vi "clump to runtime maps.vi"(4 "output dictionary":refnum<class "data dictionary.lvclass">, 6 "input dictionary":refnum<class "data dictionary.lvclass">, 7 "modbus channels":refnum<class "Modbus Module Channel.lvclass">[](array[class]), 8 "error in":errorcluster, 11 "clumps":T1[](array[typedef])) -> (0 "error out":errorcluster, 2 "output accesses":T7[](array[typedef]), 3 "input accesses":T4[](array[typedef]))   [LabVIEW 2013, in "Modbus Slave runtime.lvclass"]
uses:
  Modbus Slave runtime.lvclass
  output bulk data access.ctl
  module channel/data bank type.ctl
  data mapping elements.ctl
  <vilib>/NI/Tag Bus/tag/Data Type.ctl
  bulk data access.ctl
  module channel/Modbus Module Channel.lvclass
  <vilib>/NI/Tag Bus/dictionary/data dictionary.lvclass
  clump.ctl
  <vilib>/NI/Tag Bus Module Framework/channel/channel classification.ctl
  <vilib>/NI/Tag Bus/tag/tag descriptor.lvclass/tag descriptor.ctl
  module channel/Modbus Module Channel.lvclass/Modbus Module Channel.ctl
  <vilib>/NI/Tag Bus/tag/read data type.vi
  module channel/Read starting address.vi
  module channel/Read subindex (bool).vi
  <vilib>/NI/Tag Bus/tag/read tag name.vi
  <vilib>/NI/Tag Bus/dictionary/locate tag.vi
  <vilib>/NI/Tag Bus/tag/tag descriptor.lvclass
  <vilib>/NI/Tag Bus Module Framework/channel/TBM channel.lvclass
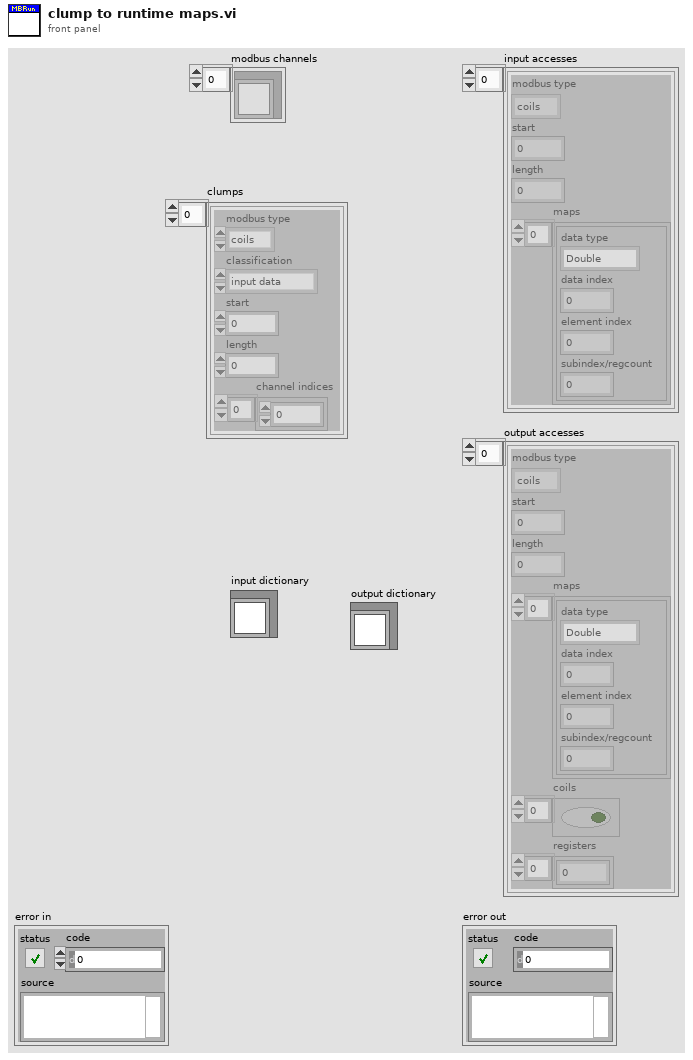
[diagram p1: front panel]
types:
  T1 = typedef "Modbus Slave runtime.lvclass/clump.ctl" = cluster{"modbus type":T2, "classification":T3, "start":i32, "length":i32, "channel indices":i32[]}
  T2 = typedef "Modbus Module Channel.lvclass/data bank type.ctl" = enum16{"coils", "discrete inputs", "input registers", "holding registers"}
  T3 = typedef "TBM channel.lvclass/channel classification.ctl" = enum16{"input data", "output data", "processing parameter", "processing result"}
  T4 = typedef "Modbus Slave runtime.lvclass/bulk data access.ctl" = cluster{"modbus type":T2, "start":u16, "length":u16, "maps":T5[]}
  T5 = typedef "Modbus Slave runtime.lvclass/data mapping elements.ctl" = cluster{"data type":T6, "data index":i32, "element index":i32, "subindex/regcount":i32}
  T6 = typedef "tag bus.lvlib/tag descriptor.lvclass/Data Type.ctl" = enum16{"Double", "Single", "I64", "I32", "I16", "I8", "U64", "U32", "U16", "U8", "Boolean", "String", "Array of Double", "Array of Single", "Array of I64", "Array of I32", "Array of I16", "Array of I8", "Array of U64", "Array of U32", "Array of U16", "Array of U8", "Array of Boolean", "Array of String"}
  T7 = typedef "Modbus Slave runtime.lvclass/output bulk data access.ctl" = cluster{"modbus type":T2, "start":u16, "length":u16, "maps":T5[], "coils":bool[], "registers":u16[]}
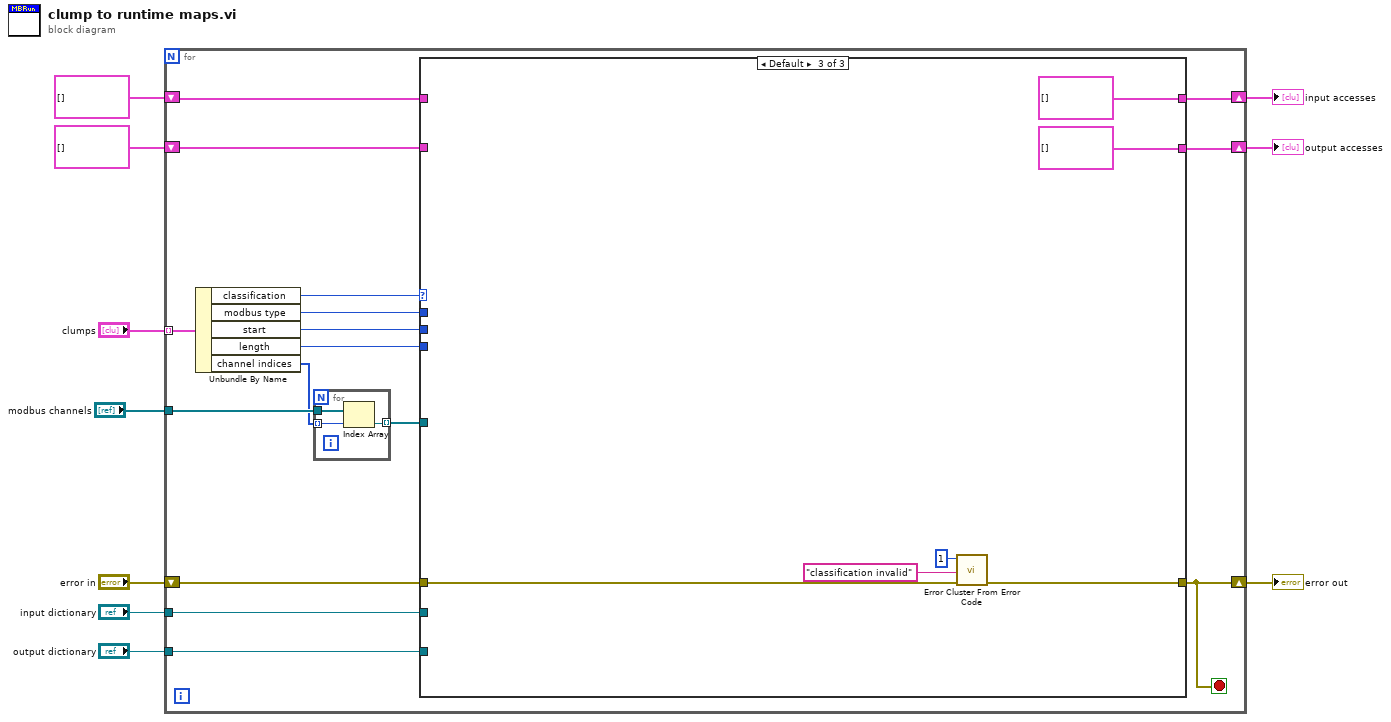
[diagram p0: block diagram]
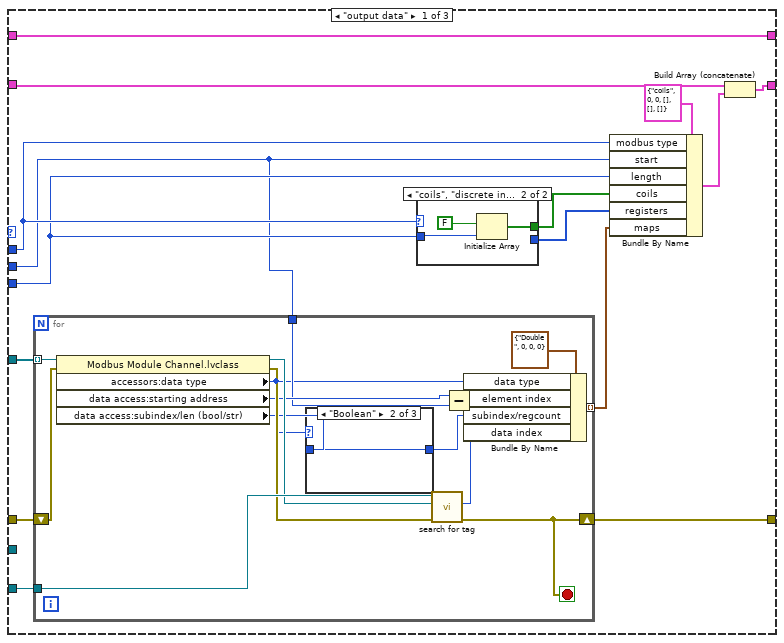
[diagram p2: hidden frame]
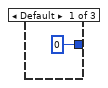
[diagram p3: hidden frame]
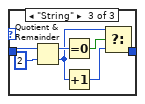
[diagram p4: hidden frame]
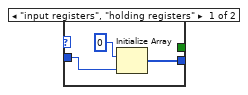
[diagram p5: hidden frame]
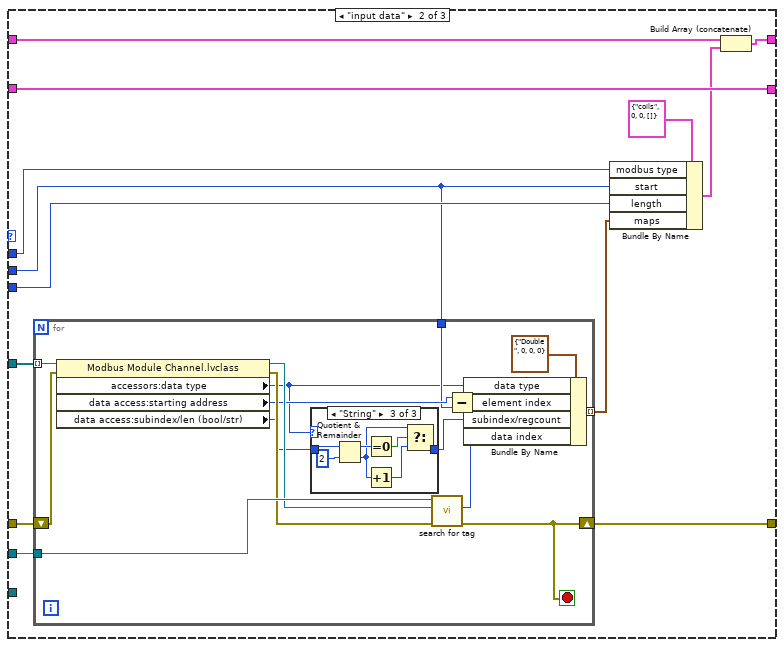
[diagram p6: hidden frame]
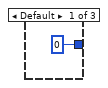
[diagram p7: hidden frame]
diagram:
  n1 = for {
    tunnel: "clumps" -> [w26] mode=indexing
    shift-right: [w20] -> w8
    shift-left: "error in" -> [w21]
    tunnel: "modbus channels" -> [w25]
    shift-right: [w22] -> w3
    shift-left: T4[] [] ("input accesses") -> [w18]
    shift-right: [w23] -> w4
    shift-left: T7[] [] ("output accesses") -> [w19]
    tunnel: "input dictionary" -> [w17]
    tunnel: "output dictionary" -> [w16]
    stop <- w20 stop-if-true
    n2 = Unbundle By Name(w26) -> ("classification"=w24:T3, "modbus type"=w15:T2, "start"=w14:i32, "length"=w13:i32, "channel indices"=w12:i32[])
    n3 = for {
      tunnel: w25 -> [w117]
      tunnel: w12 -> [w116] mode=indexing
      tunnel: [w115] -> w11 mode=indexing
      n4 = Index Array(array=w117, index=w116) -> (element=w115:refnum<class "Modbus Module Channel.lvclass">)
    }
    n5 = case shown="Default" w24 {
      tunnel: [w39 w83 T7[] [] ("output accesses")] -> w23
      tunnel: [w41 w76 T4[] [] ("input accesses")] -> w22
      tunnel: [w30 w79 w111] -> w20
      tunnel: w21 -> [w32 w80 w112]
      tunnel: w19 -> [w40 w83 _]
      tunnel: w18 -> [w41 w84 _]
      tunnel: w17 -> [_ w73 _]
      tunnel: w16 -> [w31 _ _]
      tunnel: w15 -> [w36 w82 _]
      tunnel: w14 -> [w27 w72 _]
      tunnel: w13 -> [w35 w81 _]
      tunnel: w11 -> [w28 w77 _]
      frame "output data" {
        n6 = for {
          shift-right: [w48] -> w30
          shift-left: w32 -> [w53]
          tunnel: w31 -> [w52]
          tunnel: [w55] -> w29 mode=indexing
          tunnel: w28 -> [w54] mode=indexing
          tunnel: w27 -> [w45]
          stop <- w48 stop-if-true
          n7 = property class="Modbus Module Channel.lvclass"(reference=w54, error in=w53) -> (reference out=w51:refnum<class "Modbus Module Channel.lvclass">, error out=w49:errorcluster, "accessors:data type"=w44:T6, "data access:starting address"=w46:u16, "data access:subindex/len (bool/str)"=w43:i32)
          n8 = case shown="\"Boolean\"" w44 {
            tunnel: w43 -> [_ w58 w59]
            tunnel: [0 ("data access:subindex/len (bool/str)") w58 w60] -> w42
            frame Default {
            }
            frame "Boolean" {
            }
            frame "String" {
              n9 = Quotient & Remainder(x=w59, y=2) -> (x-y*floor(x/y)=w64:i32, floor(x/y)=w62:i32)
              n10 = Equal To 0?(x=w64) -> (x = 0?=w63:bool)
              n11 = Increment(x=w62) -> (x+1=w61:i32)
              n12 = Select(t=w62, s=w63, f=w61) -> (s? t:f=w60:i32)
            }
          }
          n13 = call <vilib>:"search for tag.vi"("error in"=w49, "system tag"=w51, "data dictionary in"=w52) -> ("error out"=w48:errorcluster, "index"=w50:i32)  [unwired: 6 in, 1 out]
          n14 = Subtract(x=w46, y=w45) -> (x-y=w47:i32)
          n15 = Bundle By Name(cluster=T5 {"data type"=enum."Double", "data index"=0, "element index"=0, "subindex/regcount"=0} ("mapping element"), "data type"=w44, "element index"=w47, "subindex/regcount"=w42, "data index"=w50) -> (w55:T5)
        }
        n16 = case shown="\"coils\", \"discrete inputs\"" w36 {
          tunnel: w35 -> [w66 w71]
          tunnel: [_ w69] -> w34
          tunnel: [w68 _] -> w33
          frame "input registers", "holding registers" {
            n17 = Initialize Array(u16 0, w66) -> (w68:u16[])
          }
          frame "coils", "discrete inputs" {
            n18 = Initialize Array(FALSE, w71) -> (w69:bool[])
          }
        }
        n19 = Bundle By Name(cluster=T7 {"modbus type"=enum."coils", "start"=0, "length"=0, "maps"=[], "coils"=[], "registers"=[]} ("output data access"), "modbus type"=w36, "start"=w27, "length"=w35, "coils"=w34, "registers"=w33, "maps"=w29) -> (w37:T7)
        n20 = Build Array (concatenate)(w40, w37) -> (w39:T7[])
      }
      frame "input data" {
        n21 = for {
          shift-right: [w91] -> w79
          shift-left: w80 -> [w96]
          tunnel: w73 -> [w95]
          tunnel: [w98] -> w78 mode=indexing
          tunnel: w77 -> [w97] mode=indexing
          tunnel: w72 -> [w88]
          stop <- w91 stop-if-true
          n22 = property class="Modbus Module Channel.lvclass"(reference=w97, error in=w96) -> (reference out=w94:refnum<class "Modbus Module Channel.lvclass">, error out=w92:errorcluster, "accessors:data type"=w87:T6, "data access:starting address"=w89:u16, "data access:subindex/len (bool/str)"=w86:i32)
          n23 = case shown="\"String\"" w87 {
            tunnel: w86 -> [_ w101 w102]
            tunnel: [0 ("data access:subindex/len (bool/str)") w101 w103] -> w85
            frame Default {
            }
            frame "Boolean" {
            }
            frame "String" {
              n24 = Quotient & Remainder(x=w102, y=2) -> (x-y*floor(x/y)=w107:i32, floor(x/y)=w105:i32)
              n25 = Equal To 0?(x=w107) -> (x = 0?=w106:bool)
              n26 = Increment(x=w105) -> (x+1=w104:i32)
              n27 = Select(t=w105, s=w106, f=w104) -> (s? t:f=w103:i32)
            }
          }
          n28 = call <vilib>:"search for tag.vi"("error in"=w92, "system tag"=w94, "data dictionary in"=w95) -> ("error out"=w91:errorcluster, "index"=w93:i32)  [unwired: 6 in, 1 out]
          n29 = Subtract(x=w89, y=w88) -> (x-y=w90:i32)
          n30 = Bundle By Name(cluster=T5 {"data type"=enum."Double", "data index"=0, "element index"=0, "subindex/regcount"=0} ("mapping element"), "data type"=w87, "element index"=w90, "subindex/regcount"=w85, "data index"=w93) -> (w98:T5)
        }
        n31 = Bundle By Name(cluster=T4 {"modbus type"=enum."coils", "start"=0, "length"=0, "maps"=[]} ("bulk data access"), "modbus type"=w82, "start"=w72, "length"=w81, "maps"=w78) -> (w75:T4)
        n32 = Build Array (concatenate)(w84, w75) -> (w76:T4[])
      }
      frame Default {
        n33 = call <vilib>:"Error Cluster From Error Code.vi"("error in (no error)"=w112, "error message (\"\")"="classification invalid" ("error message (\"\")"), "error code (0)"=1) -> ("error out"=w111:errorcluster)  [unwired: 6 in]
      }
    }
  }
  "output accesses" <- w4
  "input accesses" <- w3
  "error out" <- w8
